vi "Build Plot legend.vi"(10 "Reference Values":string[](array[string]), 11 "Display Names":string[](array[string])) -> (2 "Array":bool[](array[boolean]), 3 "Plot legend Names":string[](array[string]))   [LabVIEW 2013]
doc: "This vi gives output of array with references fro variable available or not\nInput\n1. Display names\n2. References values\noutput\n1. Boolean Array"
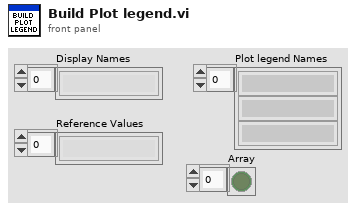
[diagram p1: front panel]
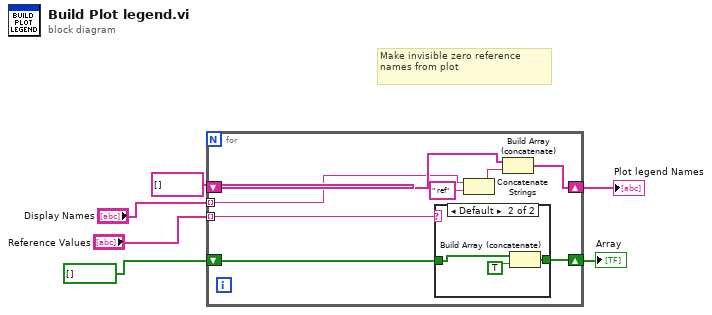
[diagram p0: block diagram]
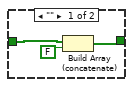
[diagram p2: hidden frame]
diagram:
  # "Make invisible zero reference names from plot"
  n1 = for {
    shift-right: [w8] -> w4
    shift-left: string[] [] -> [w9]
    tunnel: "Reference Values" -> [w14] mode=indexing
    tunnel: "Display Names" -> [w7] mode=indexing
    shift-right: [w12] -> w1
    shift-left: bool[] [] -> [w13]
    n2 = case shown="Default" w14 {
      tunnel: w13 -> [w16 w20]
      tunnel: [w15 w18] -> w12
      frame "" {
        n3 = Build Array (concatenate)(w16, FALSE) -> (w15:bool[])
      }
      frame Default {
        n4 = Build Array (concatenate)(w20, TRUE) -> (w18:bool[])
      }
    }
    n5 = Concatenate Strings(w7, " ref" ("string")) -> (w10:string)
    n6 = Build Array (concatenate)(w9, w10) -> (w8:string[])
  }
  "Plot legend Names" <- w4
  "Array" <- w1
